vi "tcp_服务器_发送.vi"(9 "远程端口或服务名称":u16=6314, 10 "原文件路径（使用对话框）":path=path "C:/Users/Administrator.2W964MZOGI5HE3B/Desktop/labview图片/105256rhad11pc5553vz5e.png", 11 "服务器网络地址":string="127.0.0.1") -> ()   [LabVIEW 2016, in "数据传输系统-02.lvlib" / "自动更新.lvlib" / "TCP文件传输系统.lvlib" / "TCP发送文件.lvlib"]
panel:
  out "长度":i32
  out "当前步骤":T1(ring)
  out "error out":errorcluster
  out "错误输出":errorcluster
  out "已传百分比":string
  out "运行指示灯":bool
  in  "分帧数(兆)":i64=2
  out "侦数":i32
  out "已发帧数":i32
  out "在发第几次":i32
  out "共发送次数":string
  in  "分一包（兆）":i64=40
  out "文件名称":string
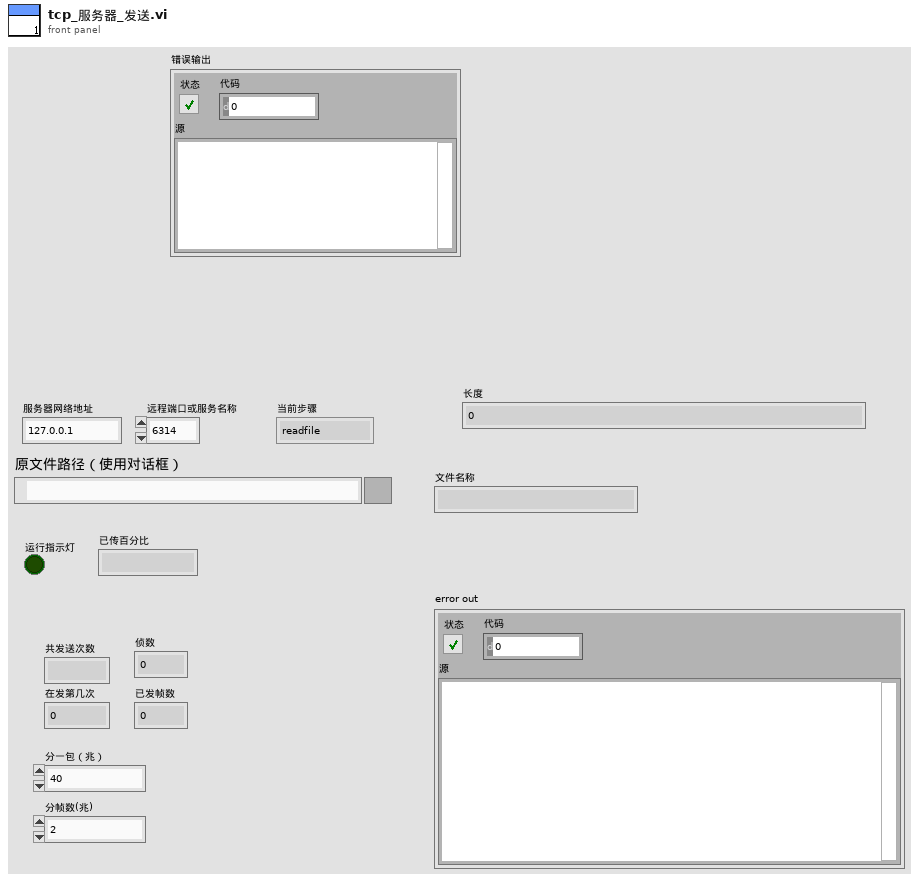
[diagram p1: front panel]
types:
  T1 = enum16{"readfile", "init", "sendhead", "sendcontent", "sendsuccess", "over"}
  T2 = enum16{"open", "replace", "create", "open or create", "replace or create", "replace or create with confirmation"}
  T3 = cluster{"网络灯":bool, "发送中":bool, "已发送百分比":u8, "发送成功次数":dbl, "当前步骤":enum16{"readfile", "init", "sendhead", "sendcontent", "sendsuccess", "over"}, "文件名":string, "error out":errorcluster}
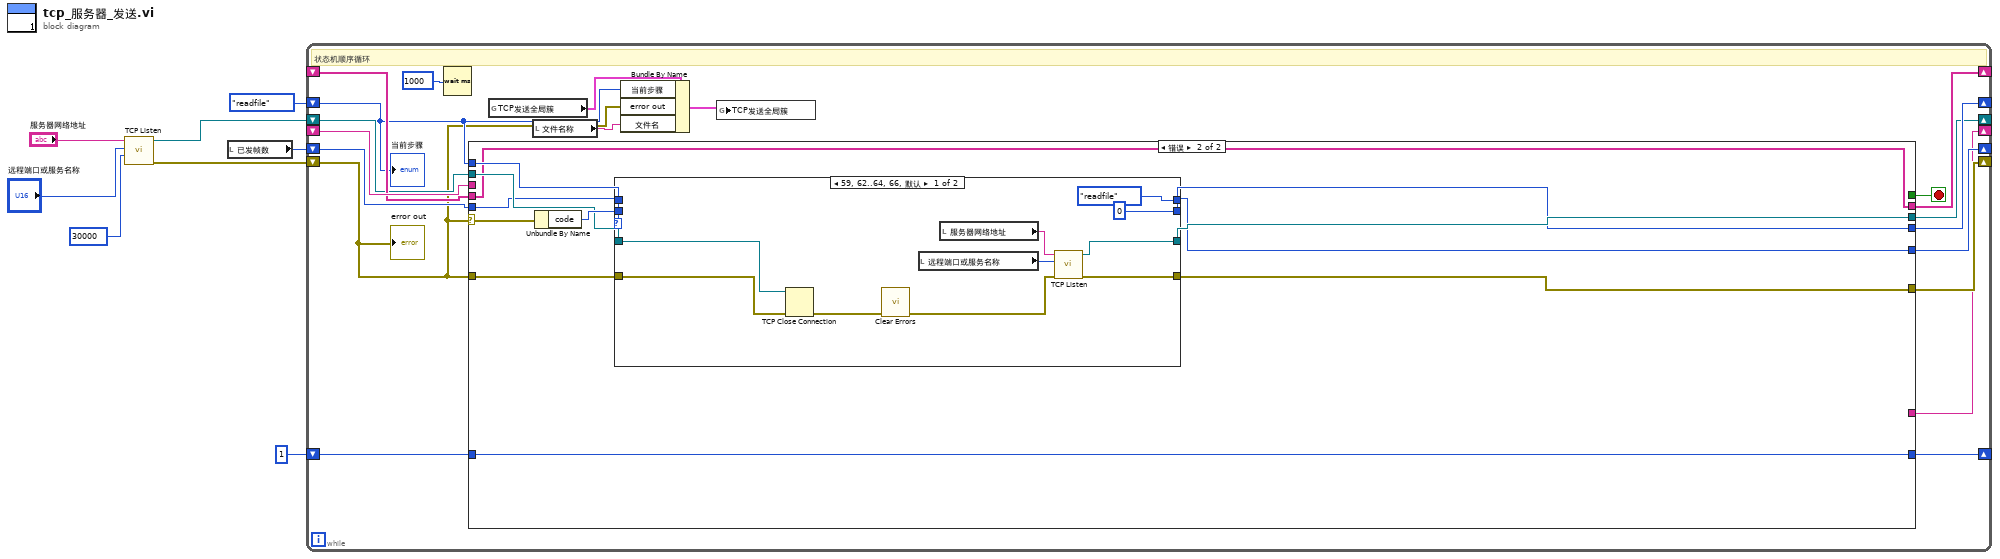
[diagram p0: block diagram]
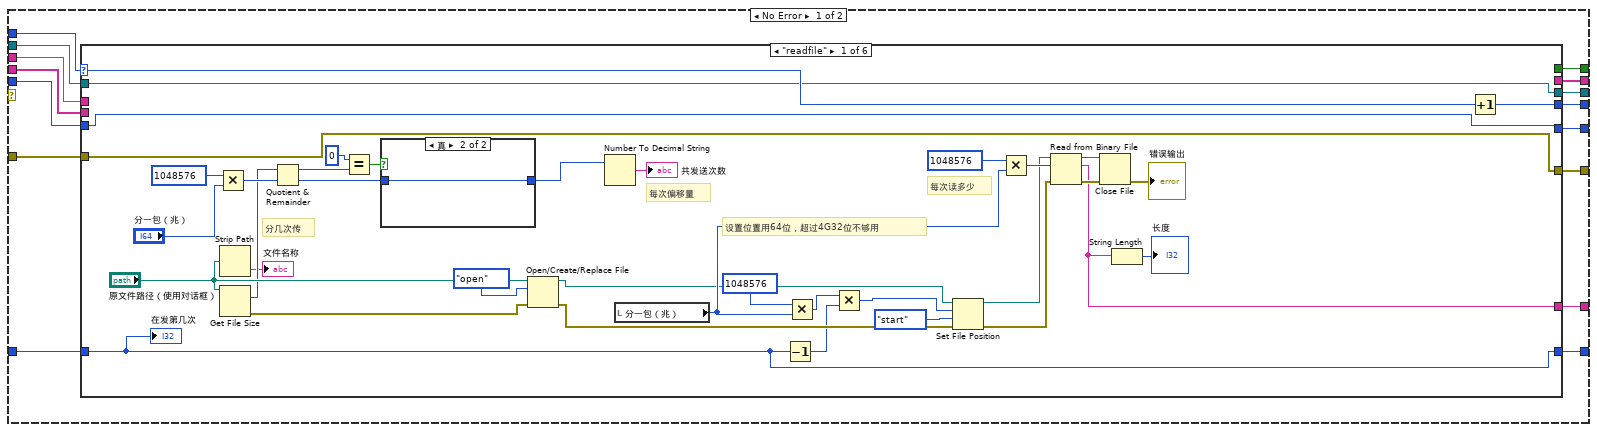
[diagram p2: hidden frame]
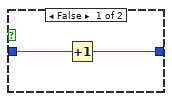
[diagram p3: hidden frame]
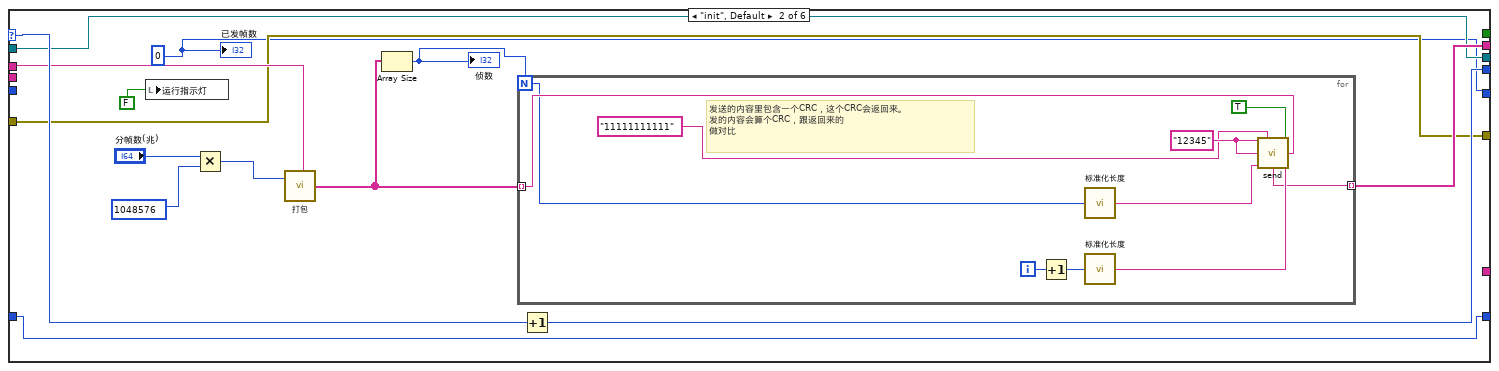
[diagram p4: hidden frame]
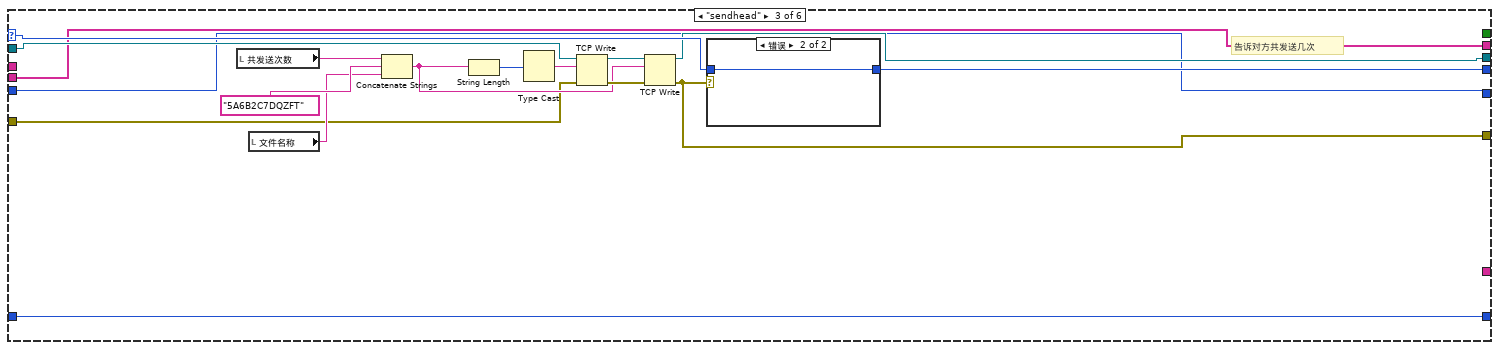
[diagram p5: hidden frame]
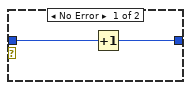
[diagram p6: hidden frame]
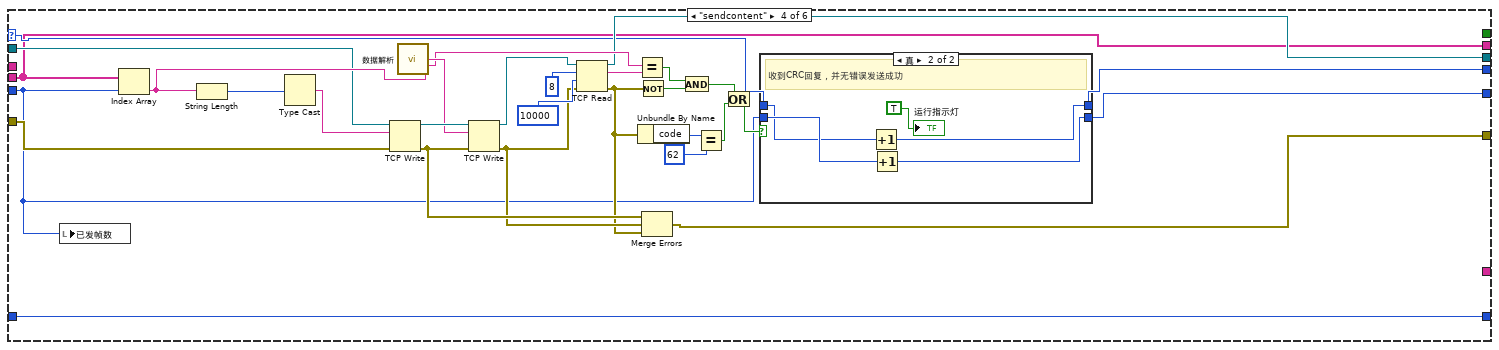
[diagram p7: hidden frame]
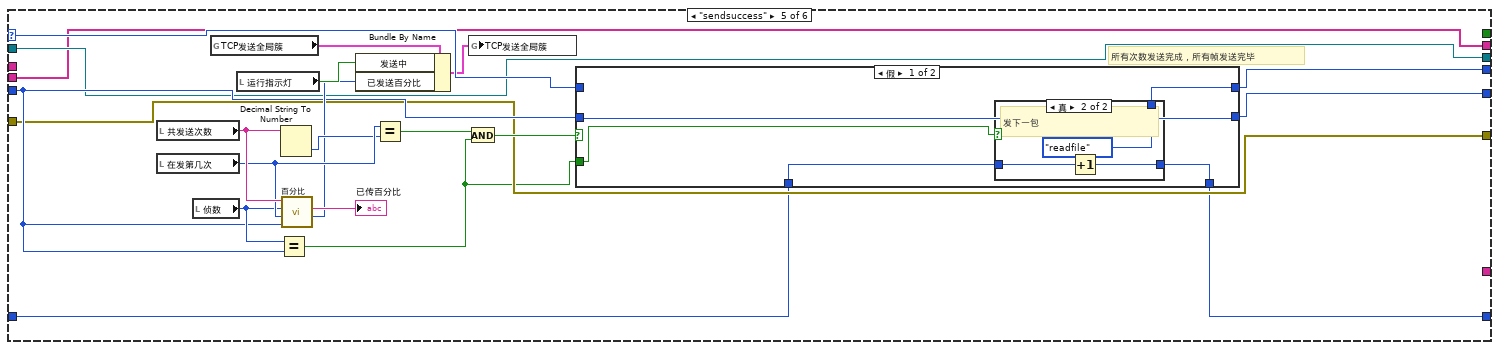
[diagram p9: hidden frame]
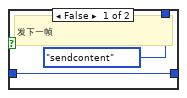
[diagram p10: hidden frame]
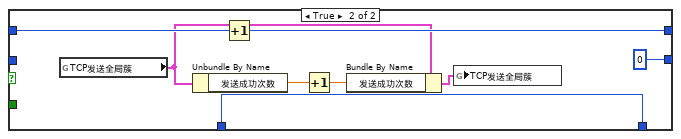
[diagram p11: hidden frame]
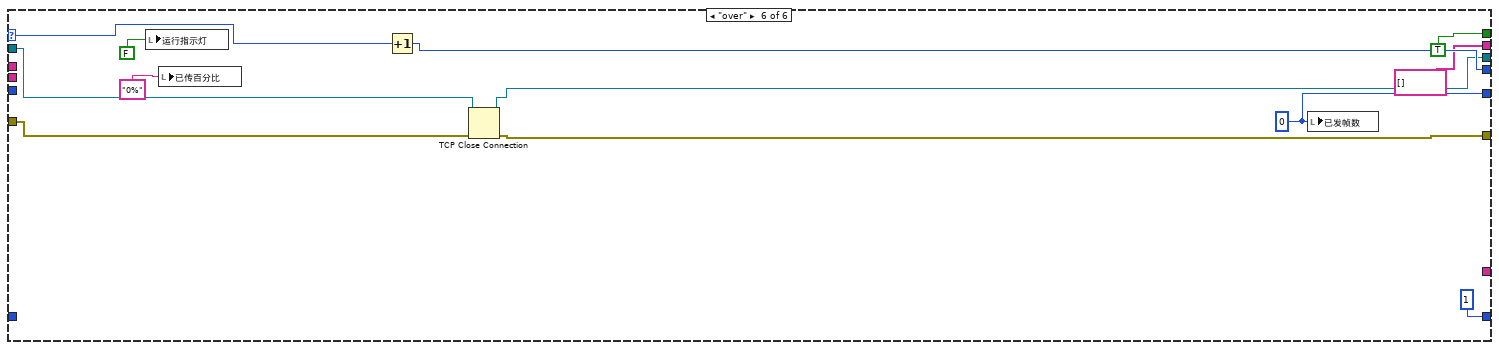
[diagram p12: hidden frame]
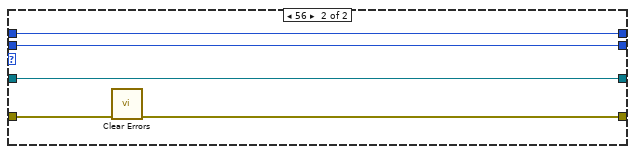
[diagram p13: hidden frame]
diagram:
  n1 = call <vilib>:"TCP Listen.vi"("timeout ms (wait forever: -1)"=30000, "port"="远程端口或服务名称", "service name"="服务器网络地址") -> ("error out"=w6:errorcluster, "connection ID"=w7:refnum<k5>)  [unwired: 4 in, 3 out]
  n2 = local read "已发帧数"() -> (w2:i32)
  n3 = while {
    shift-right: [w27] -> _
    shift-left: T1."readfile" -> [w14]
    shift-right: [w22] -> _
    shift-left: w6 -> [w13]
    shift-right: [w25] -> _
    shift-left: _ -> [w21]
    shift-right: [w19] -> _
    shift-left: w2 -> [w20]
    shift-right: [w23] -> _
    shift-left: w7 -> [w18]
    shift-right: [w11] -> _
    shift-left: _ -> [w24]
    shift-right: [w9] -> _
    shift-left: 1 ("timeout ms (wait forever: -1)") -> [w10]
    stop <- w26 stop-if-true
    # "状态机顺序循环"
    n4 = Wait (ms)(milliseconds to wait=u32 1000 ("等待时间（毫秒）")) -> ()  [unwired: 1 out]
    n5 = case shown="错误" w13 {
      selector: w13 -> [_ w226]
      tunnel: w14 -> [w42 w220]
      tunnel: [w41 w219] -> w27
      tunnel: [w40 _] -> w26
      tunnel: [w39 w218] -> w25
      tunnel: w24 -> [w38 _]
      tunnel: w13 -> [w36 w224]
      tunnel: w18 -> [w37 w223]
      tunnel: [w33 w222] -> w23
      tunnel: [w34 w221] -> w22
      tunnel: w21 -> [w35 w218]
      tunnel: w20 -> [w32 w217]
      tunnel: [w31 w216] -> w19
      tunnel: [w30 _] -> w11
      tunnel: w10 -> [w29 w215]
      tunnel: [w28 w215] -> w9
      frame No Error {
        n6 = case shown="\"readfile\"" w42 {
          selector: w42 -> [w78 w96 w123 w136 w184 w214]
          tunnel: [w79 w95 w122 w135 w183 w213] -> w41
          tunnel: [_ _ _ _ _ TRUE] -> w40
          tunnel: [_ w89 w111 w134 w167 string[] []] -> w39
          tunnel: w38 -> [_ w88 _ _ _ _]
          tunnel: w37 -> [w50 w87 w113 w141 w169 w210]
          tunnel: w36 -> [w43 w86 w112 w142 w168 w209]
          tunnel: w35 -> [_ _ w111 w134 w167 _]
          tunnel: [w43 w86 w108 w139 w168 w207] -> w34
          tunnel: [w50 w87 w110 w140 w169 w208] -> w33
          tunnel: w32 -> [w49 _ w109 w127 w170 _]
          tunnel: [w49 w83 w109 w137 w171 w211] -> w31
          tunnel: [w46 _ _ _ _ _] -> w30
          tunnel: w29 -> [w47 w84 w107 w128 w166 _]
          tunnel: [w47 w84 w107 w128 w165 1 ("timeout ms (wait forever: -1)")] -> w28
          frame "readfile" {
            # "设置位置用64位，超过4G32位不够用"
            # "每次读多少"
            # "每次偏移量"
            # "分几次传"
            n7 = Multiply(x=i64 1048576 ("y"), y="分一包（兆）") -> (x*y=w76:i64)
            n8 = Strip Path(path="原文件路径（使用对话框）") -> (name=→"文件名称":string)  [unwired: 1 out]
            n9 = Get File Size(file="原文件路径（使用对话框）") -> (size (in bytes)=w72:i64, 0:w71:errorcluster)  [unwired: 1 in, 1 out]
            n10 = Quotient & Remainder(x=w72, y=w76) -> (x-y*floor(x/y)=w67:i64, floor(x/y)=w70:i64)
            n11 = Equal?(x=0, y=w67) -> (x = y?=w69:bool)
            n12 = case shown="真" w69 {
              tunnel: [w80 w82] -> w53
              tunnel: w70 -> [w81 w82]
              frame False {
                n13 = Increment(x=w81) -> (x+1=w80:i64)
              }
              frame True {
              }
            }
            n14 = Open/Create/Replace File(file path (use dialog)="原文件路径（使用对话框）", error in=w71, operation (0:open)=T2."open" ("操作(0:open)")) -> (refnum out=w52:refnum<file>, error out=w51:errorcluster)  [unwired: 3 in, 1 out]
            n15 = Number To Decimal String(number=w53) -> (decimal integer string=→"共发送次数":string)  [unwired: 1 in]
            n16 = local read "分一包（兆）"() -> (w63:i64)
            n17 = Decrement(x=w47) -> (x-1=w48:i32)
            n18 = Multiply(x=i64 1048576 ("偏移量（字节）（0）"), y=w63) -> (x*y=w60:i64)
            n19 = Multiply(x=w60, y=w48) -> (x*y=w58:i64)
            n20 = Set File Position(offset (in bytes) (0)=w58, refnum=w52, from (0:start)=enum16{"start", "end", "current"}."start" ("自（0:起始）"), error in=w51) -> (refnum out=w56:refnum<file>, error out=w55:errorcluster)
            n21 = Multiply(x=1048576 ("总数(1)"), y=w63) -> (x*y=w62:i64)
            n22 = Read from Binary File(8:w55, 10:w62, 11:w56) -> (0:w65:errorcluster, 2:w46:string, 3:w64:refnum<file>)  [unwired: 3 in, 1 out]
            n23 = Close File(refnum=w64, error in=w65) -> (error out=→"错误输出":errorcluster)  [unwired: 1 out]
            n24 = String Length(string=w46) -> (length=→"长度":i32)
            n25 = Increment(x=w78) -> (x+1=w79:T1)
            "在发第几次" <- w47
          }
          frame "init", Default {
            w83 = 0 ("数值")
            n26 = local write "运行指示灯"(FALSE ("运行指示灯")) -> ()
            n27 = Multiply(x="分帧数(兆)", y=i64 1048576) -> (x*y=w93:i64)
            n28 = call "打包.vi"("总内容"=w88, "分包大小"=w93) -> ("分包数组"=w92:string[])
            n29 = Array Size(array=w92) -> (size(s)=w94:i32)
            "侦数" <- w94
            n30 = for {
              N: w94 -> [w101]
              tunnel: w92 -> [w106] mode=indexing
              tunnel: [w99] -> w89 mode=indexing
              i -> [w105]
              w98 = "12345" ("内容说明（文件名）")
              # "发送的内容里包含一个CRC，这个CRC会返回来。\n发的内容会算个CRC，跟返回来的\n做对比"
              n31 = Increment(x=w105) -> (x+1=w100:i32)
              n32 = call "标准化长度.vi"("原长度"=w101) -> ("标准化长度"=w104:string)
              n33 = call "标准化长度.vi"("原长度"=w100) -> ("标准化长度"=w103:string)
              n34 = call "send.vi"("内容标识"=w98, "时标"="11111111111", "发送"=TRUE, "内容说明（文件名）"=w98, "帧内容"=w106, "帧数"=w104, "帧号"=w103) -> ("连接的字符串"=w99:string)  [unwired: 6 in, 2 out]
            }
            n35 = Increment(x=w96) -> (x+1=w95:T1)
            "已发帧数" <- w83
          }
          frame "sendhead" {
            # "告诉对方共发送几次"
            n36 = local read "共发送次数"() -> (w118:string)
            n37 = local read "文件名称"() -> (w119:string)
            n38 = Concatenate Strings(w118, "5A6B2C7DQZFT" ("字符串"), w119) -> (w114:string)
            n39 = String Length(string=w114) -> (length=w121:i32)
            n40 = Type Cast(x=w121) -> (*(type *) &x=w115:string)  [unwired: 1 out]
            n41 = TCP Write(connection ID=w113, data in=w115, error in (no error)=w112) -> (connection ID out=w116:refnum<k5>, error out=w117:errorcluster)  [unwired: 2 out]
            n42 = TCP Write(connection ID=w116, data in=w114, error in (no error)=w117) -> (connection ID out=w110:refnum<k5>, error out=w108:errorcluster)  [unwired: 2 out]
            n43 = case shown="错误" w108 {
              tunnel: w123 -> [w125 w126]
              tunnel: [w124 w126] -> w122
              frame No Error {
                n44 = Increment(x=w125) -> (x+1=w124:T1)
              }
              frame Error {
              }
            }
          }
          frame "sendcontent" {
            n45 = local write "已发帧数"(w127) -> ()
            n46 = Index Array(array=w134, index=w127) -> (element=w151:string)
            n47 = String Length(string=w151) -> (length=w155:i32)
            n48 = Type Cast(x=w155) -> (*(type *) &x=w152:string)  [unwired: 1 out]
            n49 = TCP Write(connection ID=w141, data in=w152, error in (no error)=w142) -> (connection ID out=w156:refnum<k5>, error out=w144:errorcluster)  [unwired: 2 out]
            n50 = call "数据解析.vi"("data in"=w151) -> ("data out"=w150:string, "CRC"=w148:string)  [unwired: 4 in, 9 out]
            n51 = TCP Write(connection ID=w156, data in=w150, error in (no error)=w144) -> (connection ID out=w154:refnum<k5>, error out=w143:errorcluster)  [unwired: 2 out]
            n52 = TCP Read(connection ID=w154, bytes to read=8 ("读取的字节"), error in (no error)=w143, 9:10000 ("超时毫秒(25000)")) -> (connection ID out=w140:refnum<k5>, data out=w149:string, error out=w133:errorcluster)  [unwired: 1 in]
            n53 = Equal?(x=w148, y=w149) -> (x = y?=w146:bool)
            n54 = Not(x=w133) -> (.not. x?=w145:bool)
            n55 = Unbundle By Name(w133) -> ("code"=w131:i32)
            n56 = Merge Errors(w144, w143, w133) -> (w139:errorcluster)
            n57 = And(x=w146, y=w145) -> (x .and. y?=w138:bool)
            n58 = Equal?(x=w131, y=62) -> (x = y?=w129:bool)
            n59 = Or(x=w138, y=w129) -> (x .or. y?=w132:bool)
            n60 = case shown="真" w132 {
              tunnel: w127 -> [w158 w162]
              tunnel: [w158 w161] -> w137
              tunnel: w136 -> [w157 w160]
              tunnel: [w157 w159] -> w135
              frame False {
                # "未收到正确回复，或超时"
              }
              frame True {
                # "收到CRC回复，并无错误发送成功"
                n61 = Increment(x=w160) -> (x+1=w159:T1)
                n62 = Increment(x=w162) -> (x+1=w161:i32)
                "运行指示灯" <- TRUE
              }
            }
          }
          frame "sendsuccess" {
            # "所有次数发送完成，所有帧发送完毕"
            n63 = local read "共发送次数"() -> (w181:string)
            n64 = local read "在发第几次"() -> (w180:i32)
            n65 = local read "侦数"() -> (w178:i32)
            n66 = global read "全局变量1.vi" "TCP发送全局簇"() -> (w174:T3)
            n67 = local read "运行指示灯"() -> (w173:bool)
            n68 = Equal?(x=w178, y=w170) -> (x = y?=w164:bool)
            n69 = Decimal String To Number(string=w181) -> (number=w179:i32)  [unwired: 2 in, 1 out]
            n70 = call "百分比.vi"("已发帧数 2"=w170, "发第几次"=w180, "帧数"=w178, "共发送次数"=w181) -> ("已发送百分比"=w172:u8, "已传百分比"=→"已传百分比":string)  [unwired: 6 in]
            n71 = Bundle By Name(cluster=w174, "发送中"=w173, "已发送百分比"=w172) -> (w175:T3)
            n72 = Equal?(x=w180, y=w179) -> (x = y?=w177:bool)
            n73 = And(x=w177, y=w164) -> (x .and. y?=w176:bool)
            n74 = global write "全局变量1.vi" "TCP发送全局簇"(w175) -> ()
            n75 = case shown="假" w176 {
              tunnel: w184 -> [_ w202]
              tunnel: [w187 w201] -> w183
              tunnel: [w189 0 ("已发帧数")] -> w171
              tunnel: w170 -> [w189 _]
              tunnel: w166 -> [w186 w195]
              tunnel: [w185 w195] -> w165
              tunnel: w164 -> [w188 _]
              frame False {
                n76 = case shown="真" w188 {
                  tunnel: [T1."sendcontent" T1."readfile"] -> w187
                  tunnel: w186 -> [w190 w193]
                  tunnel: [w190 w192] -> w185
                  frame False {
                    # "发下一帧"
                  }
                  frame True {
                    # "发下一包"
                    n77 = Increment(x=w193) -> (x+1=w192:i32)
                  }
                }
              }
              frame True {
                n78 = global read "全局变量1.vi" "TCP发送全局簇"() -> (w197:T3)
                n79 = Unbundle By Name(w197) -> ("发送成功次数"=w198:dbl)
                n80 = Increment(x=w202) -> (x+1=w201:T1)
                n81 = Increment(x=w198) -> (x+1=w199:dbl)
                n82 = Bundle By Name(cluster=w197, "发送成功次数"=w199) -> (w200:T3)
                n83 = global write "全局变量1.vi" "TCP发送全局簇"(w200) -> ()
              }
            }
          }
          frame "over" {
            w211 = 0
            n84 = local write "运行指示灯"(FALSE ("运行指示灯")) -> ()
            n85 = local write "已传百分比"("0%" ("已传百分比")) -> ()
            n86 = Increment(x=w214) -> (x+1=w213:T1)
            n87 = TCP Close Connection(connection ID=w210, error in (no error)=w209) -> (connection ID out=w208:refnum<k5>, error out=w207:errorcluster)  [unwired: 1 in]
            n88 = local write "已发帧数"(w211) -> ()
          }
        }
      }
      frame Error {
        n89 = Unbundle By Name(w226) -> ("code"=w225:i32)
        n90 = case shown="59, 62..64, 66, 默认" w225 {
          tunnel: w224 -> [w236 w239]
          tunnel: w223 -> [w235 w238]
          tunnel: [w233 w238] -> w222
          tunnel: [w234 w237] -> w221
          tunnel: w220 -> [_ w241]
          tunnel: [T1."readfile" w241] -> w219
          tunnel: w217 -> [_ w240]
          tunnel: [0 ("已发帧数") w240] -> w216
          frame 59, 62..64, 66, Default {
            n91 = TCP Close Connection(connection ID=w235, error in (no error)=w236) -> (error out=w232:errorcluster)  [unwired: 1 in, 1 out]
            n92 = call <vilib>:"Clear Errors.vi"("error in (no error)"=w232) -> ("error out"=w229:errorcluster)  [unwired: 5 in, 1 out]
            n93 = local read "远程端口或服务名称"() -> (w230:u16)
            n94 = local read "服务器网络地址"() -> (w231:string)
            n95 = call <vilib>:"TCP Listen.vi"("error in (no error)"=w229, "port"=w230, "service name"=w231) -> ("error out"=w234:errorcluster, "connection ID"=w233:refnum<k5>)  [unwired: 4 in, 3 out]
          }
          frame 56 {
            n96 = call <vilib>:"Clear Errors.vi"("error in (no error)"=w239) -> ("error out"=w237:errorcluster)  [unwired: 5 in, 1 out]
          }
        }
      }
    }
    n97 = global read "全局变量1.vi" "TCP发送全局簇"() -> (w16:T3)
    n98 = local read "文件名称"() -> (w12:string)
    n99 = Bundle By Name(cluster=w16, "当前步骤"=w14, "error out"=w13, "文件名"=w12) -> (w15:T3)
    n100 = global write "全局变量1.vi" "TCP发送全局簇"(w15) -> ()
    "error out" <- w13
    "当前步骤" <- w14
  }
